vi "dfd_Mth-order Chebyshev polynomial.vi"(1 "M":i32, 2 "x":dbl format="%.2f") -> (0 "CM(x)":dbl format="%.2f")   [LabVIEW 2017, in "NI_DigFilter_Design.lvlib"]
uses:
  <vilib>/addons/Digital Filter Design/NI_DigFilter_Design.lvlib
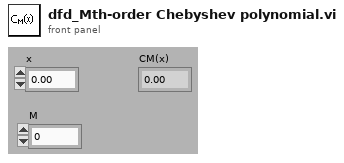
[diagram p1: front panel]
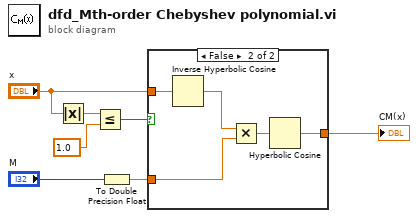
[diagram p0: block diagram]
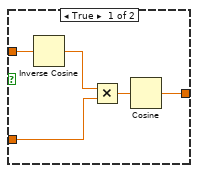
[diagram p2: hidden frame]
diagram:
  n1 = Absolute Value(x="x") -> (abs(x)=w7:dbl)
  n2 = Less Or Equal?(x=w7, y=1.0) -> (x <= y?=w5:bool)
  n3 = To Double Precision Float(number="M") -> (double precision float=w3:dbl)
  n4 = case shown="False" w5 {
    tunnel: "x" -> [w12 w17]
    tunnel: w3 -> [w10 w15]
    tunnel: [w8 w13] -> w1
    frame True {
      n5 = Inverse Cosine(1:w12) -> (0:w11:dbl)
      n6 = Multiply(x=w11, y=w10) -> (x*y=w9:dbl)
      n7 = Cosine(x=w9) -> (cos(x)=w8:dbl)
    }
    frame False {
      n8 = Inverse Hyperbolic Cosine(1:w17) -> (0:w16:dbl)
      n9 = Multiply(x=w16, y=w15) -> (x*y=w14:dbl)
      n10 = Hyperbolic Cosine(1:w14) -> (0:w13:dbl)
    }
  }
  "CM(x)" <- w1
